vi "Quiz3.vi"() -> ()   [LabVIEW 2019]
panel:
  in  "Tab Control":enum32{"User", "Admi", "DeBug"}(tab)
  out "Gráfica temperatura":dbl(graph)=50.42767726953025
  in  "Temp Max":dbl
  in  "Temp Min":dbl
  out "Alerta":string
  out "Temp Mínima":dbl
  out "Temp máxima":dbl
  in  "Temperatura C":dbl
  out "Temperatura C.":string
  out "Resistencia NTC":dbl
  out "Voltaje":dbl
  out "Temperatura F.":string="-459,670000"
  in  "TIEMPO DE GRAFIACIÓN":dbl
  in  "ALMACENAR CADA Y TIME":dbl
  in  "ADQUIRIR CADA X TIME":dbl
  in  "Escribir Warnings":bool
  in  "Escribir todos lo datos":bool
  in  "MANUAL":bool
  in  "STOP":bool=TRUE
  in  "INICIO":bool=TRUE
  out "Alerta.":string
  out "Gráfica temperatura 3":dbl(graph)=50.42767726953025
  in  "Tab  control graficas":enum32{"Datos ", "Warnings", "Gráfica"}(tab)
  in  "Datos":i32(listbox)
  in  "Warnings":i32(listbox)
  out "Gráfica temperatura 2":dbl(graph)=50.42767726953025
  out "Temperatura °C":string="-273,150000"
  out "ALERTA":string
  # "°C"
  # "°F"
  # "Ohms"
  # "V"
  # "sg"
  # "sg"
  # "sg"
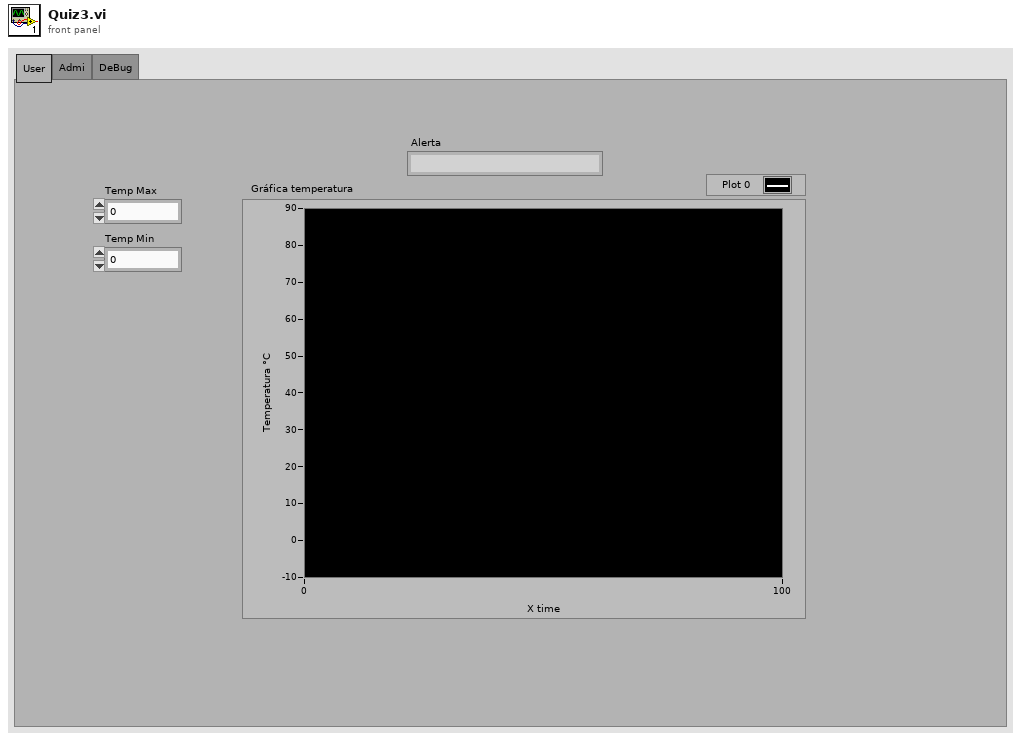
[diagram p1: front panel]
types:
  T1 = cluster{" Grados Cent.":string, "Grados Fare.":string, "date/time string":string, "Nombre del archivo txt":string}
  T2 = cluster{"Temperatura C.":string, "date/time string":string, string, "Nombre del archivo txt":string}
  T3 = cluster{" Grados Cent.":string, "Grados Fare.":string, "date/time string":string, "Nombre del archivo txt":string}[]
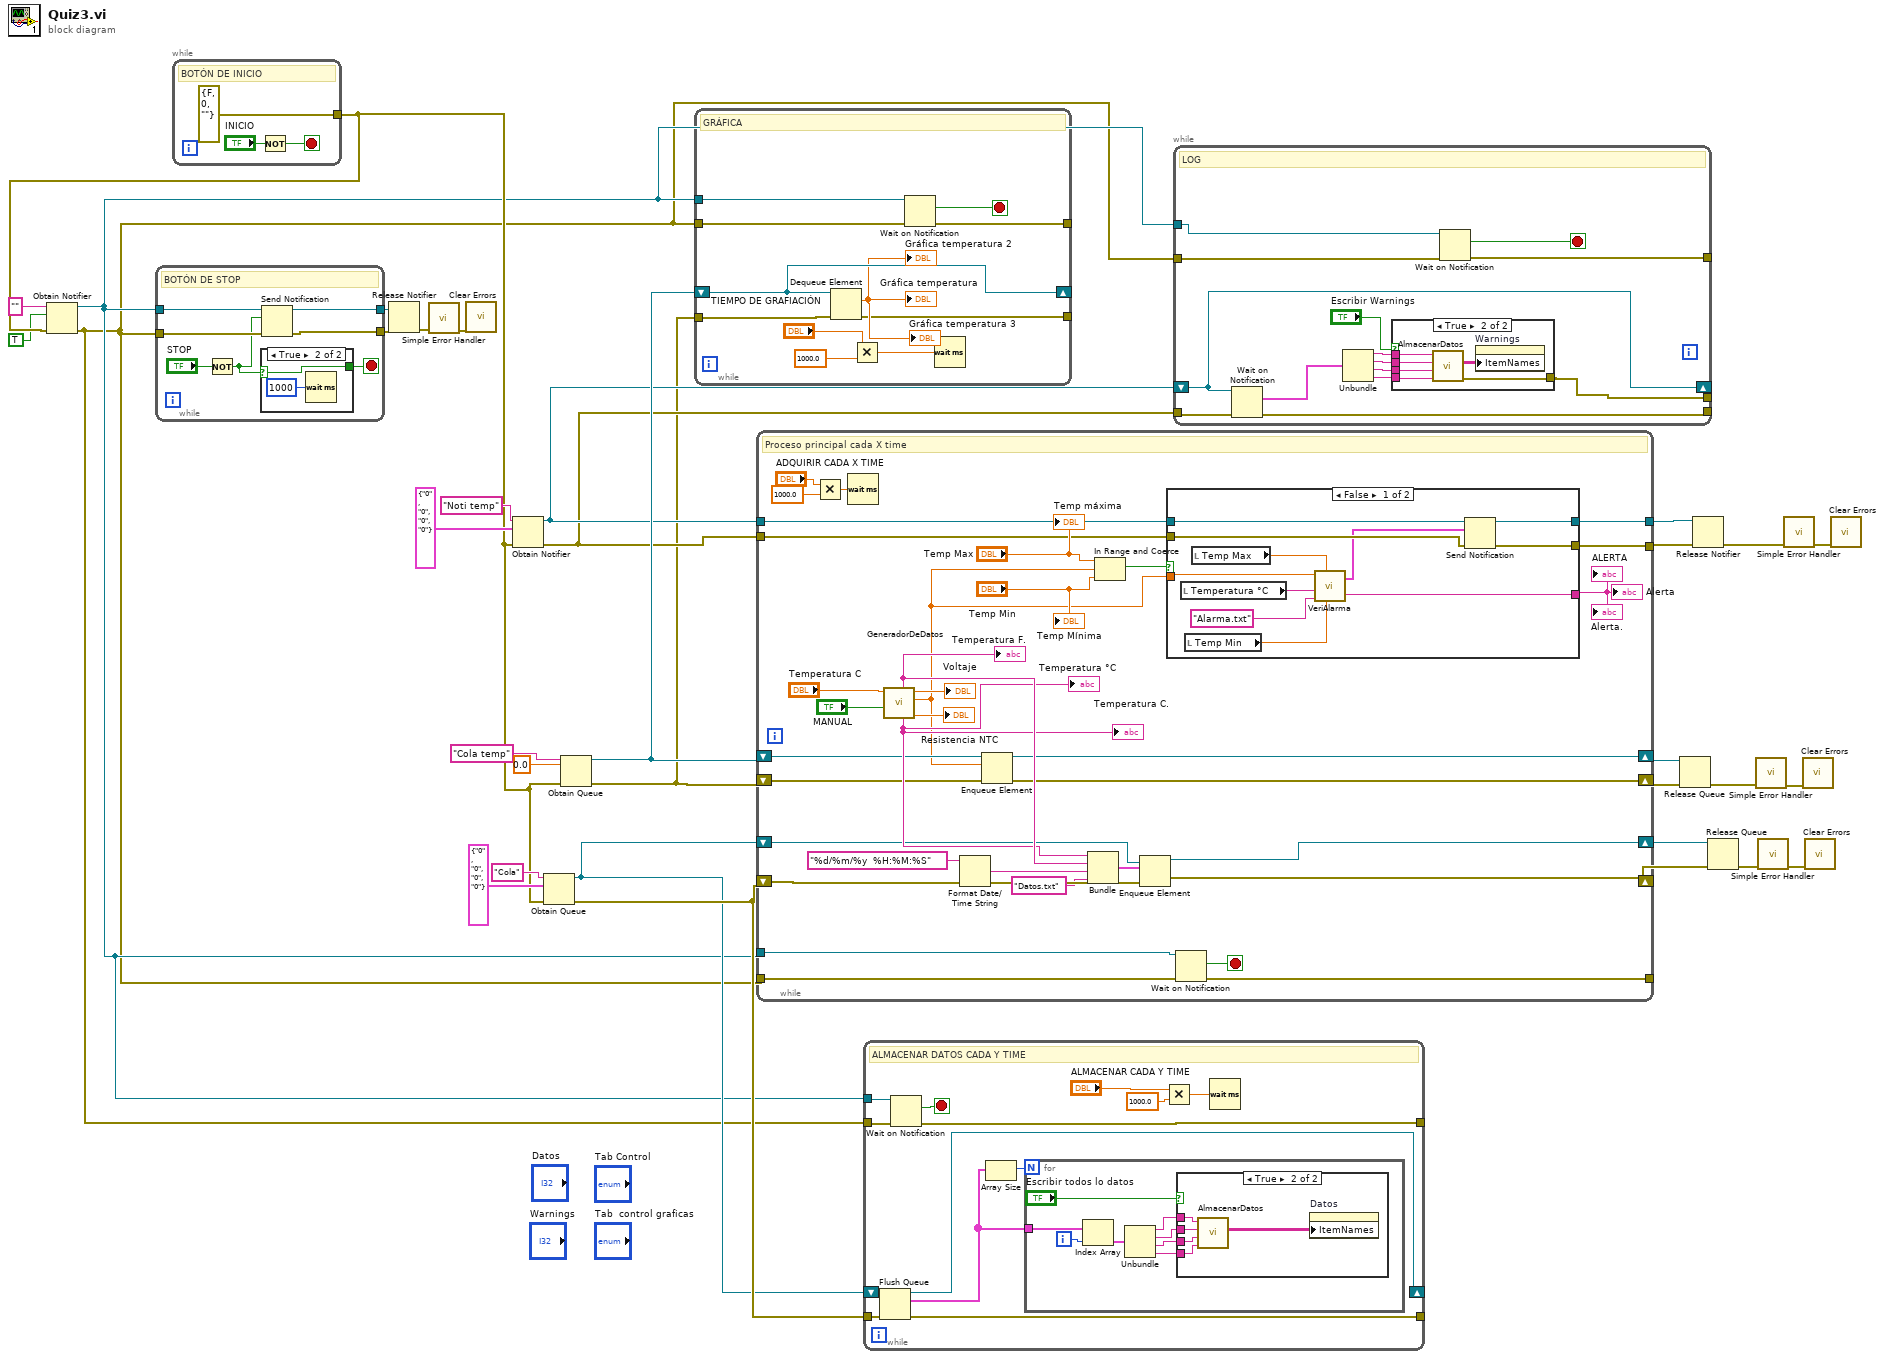
[diagram p0: block diagram]
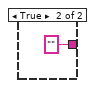
[diagram p5: hidden frame]
diagram:
  n1 = while {
    tunnel: [errorcluster {"status"=FALSE, "code"=0, "source"=""} ("error in (no error)")] -> w10
    stop <- w35 stop-if-true
    # "BOTÓN DE INICIO"
    n2 = Not(x="INICIO") -> (.not. x?=w35:bool)
  }
  n3 = Obtain Notifier(name (unnamed)="", notification data type=TRUE, error in (no error)=w10) -> (notifier out=w2:refnum<notifier>, error out=w1:errorcluster)  [unwired: 1 in, 1 out]
  n4 = while {
    tunnel: w2 -> [w42]
    tunnel: w1 -> [w41]
    tunnel: [w40] -> w6
    tunnel: [w39] -> w4
    stop <- w37 stop-if-true
    # "BOTÓN DE STOP"
    n5 = Not(x="STOP") -> (.not. x?=w38:bool)
    n6 = case shown="True" w38 {
      selector: w38 -> [_ w44]
      tunnel: [_ w44] -> w37
      frame False {
      }
      frame True {
        n7 = Wait (ms)(milliseconds to wait=u32 1000) -> ()  [unwired: 1 out]
      }
    }
    n8 = Send Notification(notification=w38, notifier=w42, error in (no error)=w41) -> (notifier out=w39:refnum<notifier>, error out=w40:errorcluster)
  }
  n9 = Release Notifier(notifier=w4, error in (no error)=w6) -> (error out=w7:errorcluster)  [unwired: 1 in, 2 out]
  n10 = call <vilib>:"Simple Error Handler.vi"("error in (no error)"=w7) -> ("error out"=w5:errorcluster)  [unwired: 4 in, 4 out]
  n11 = call <vilib>:"Clear Errors.vi"("error in (no error)"=w5) -> ()  [unwired: 5 in, 2 out]
  n12 = Obtain Notifier(name (unnamed)="Noti temp", notification data type=T1 {" Grados Cent."="0", "Grados Fare."="0", "date/time string"="0", "Nombre del archivo txt"="0"} ("output cluster"), error in (no error)=w10) -> (notifier out=w21:refnum<notifier>, error out=w20:errorcluster)  [unwired: 1 in, 1 out]
  n13 = Obtain Queue(name (unnamed)="Cola", element data type=T1 {" Grados Cent."="0", "Grados Fare."="0", "date/time string"="0", "Nombre del archivo txt"="0"} ("output cluster"), error in (no error)=w10) -> (queue out=w17:refnum<queue>, error out=w32:errorcluster)  [unwired: 2 in, 1 out]
  n14 = Obtain Queue(name (unnamed)="Cola temp", element data type=0.0, error in (no error)=w10) -> (queue out=w25:refnum<queue>, error out=w3:errorcluster)  [unwired: 2 in, 1 out]
  n15 = while {
    shift-right: [w56] -> _
    shift-left: w25 -> [w56]
    tunnel: w2 -> [w51]
    tunnel: w1 -> [w50]
    tunnel: w3 -> [w49]
    tunnel: [w48] -> _
    tunnel: [w46] -> _
    stop <- w47 stop-if-true
    # "GRÁFICA"
    n16 = Dequeue Element(queue=w56, error in (no error)=w49) -> (element=→"Gráfica temperatura" →"Gráfica temperatura 2" →"Gráfica temperatura 3":dbl, error out=w48:errorcluster)  [unwired: 1 in, 2 out]
    n17 = Multiply(x="TIEMPO DE GRAFIACIÓN", y=1000.0) -> (x*y=w54:dbl)
    n18 = Wait on Notification(notifier=w51, error in (no error)=w50) -> (notification=w47:bool, error out=w46:errorcluster)  [unwired: 2 in, 2 out]
    n19 = Wait (ms)(milliseconds to wait=w54) -> ()  [unwired: 1 out]
  }
  n20 = while {
    shift-right: [w78] -> w31
    shift-left: w17 -> [w82]
    shift-right: [w62] -> w30
    shift-left: w32 -> [w81]
    shift-right: [w75] -> w27
    shift-left: w25 -> [w77]
    shift-right: [w63] -> w26
    shift-left: w3 -> [w76]
    tunnel: w21 -> [w71]
    tunnel: [w69] -> w23
    tunnel: w20 -> [w70]
    tunnel: [w68] -> w22
    tunnel: w2 -> [w60]
    tunnel: w1 -> [w59]
    tunnel: [w57] -> _
    stop <- w58 stop-if-true
    # "Proceso principal cada X time"
    n21 = Multiply(x="ADQUIRIR CADA X TIME", y=1000.0) -> (x*y=w64:dbl)
    n22 = Wait (ms)(milliseconds to wait=w64) -> ()  [unwired: 1 out]
    n23 = call "GeneradorDeDatos.vi"("MANUAL"="MANUAL", "Temp"="Temperatura C") -> ("NTC"=→"Resistencia NTC":dbl, "Grados C graf"=w67:dbl, "Voltaje"=→"Voltaje":dbl, "Grados Cent."=w87:string, "Grados Fare."=w88:string)  [unwired: 5 in]
    "Temperatura C." <- w87
    "Temperatura F." <- w88
    "Temperatura °C" <- w87
    n24 = Format Date/Time String(time format string (%c)="%d/%m/%y  %H:%M:%S") -> (date/time string=w89:string)  [unwired: 2 in]
    n25 = Enqueue Element(queue=w77, element=w67, error in (no error)=w76) -> (queue out=w75:refnum<queue>, error out=w63:errorcluster)  [unwired: 1 in, 1 out]
    n26 = Bundle("Grados Cent."=w87, "Grados Fare."=w88, "date/time string"=w89, "Nombre del archivo txt"="Datos.txt") -> (w90:T1)  [unwired: 1 in]
    n27 = In Range and Coerce(upper limit="Temp Max", x=w67, lower limit="Temp Min") -> (In Range?=w72:bool)  [unwired: 1 out]
    n28 = Enqueue Element(queue=w82, element=w90, error in (no error)=w81) -> (queue out=w78:refnum<queue>, error out=w62:errorcluster)  [unwired: 1 in, 1 out]
    n29 = case shown="False" w72 {
      tunnel: w71 -> [w101 _]
      tunnel: w70 -> [w100 _]
      tunnel: [w99 _] -> w69
      tunnel: [w98 _] -> w68
      tunnel: w67 -> [w91 _]
      tunnel: [w96 ""] -> w66
      frame False {
        n30 = local read "Temperatura °C"() -> (w93:string)
        n31 = local read "Temp Min"() -> (w94:dbl)
        n32 = local read "Temp Max"() -> (w95:dbl)
        n33 = call "VeriAlarma.vi"("Temp Min"=w94, "Temp Max"=w95, "Nombre del archivo txt"="Alarma.txt", "Temp grados C"=w93, "Grados C"=w91) -> ("Alarma"=w96:string, "Notify Datos"=w97:T2)  [unwired: 1 in]
        n34 = Send Notification(notification=w97, notifier=w101, error in (no error)=w100) -> (notifier out=w99:refnum<notifier>, error out=w98:errorcluster)
      }
      frame True {
      }
    }
    "Alerta" <- w66
    "ALERTA" <- w66
    "Alerta." <- w66
    n35 = Wait on Notification(notifier=w60, error in (no error)=w59) -> (notification=w58:bool, error out=w57:errorcluster)  [unwired: 2 in, 2 out]
    "Temp Mínima" <- "Temp Min"
    "Temp máxima" <- "Temp Max"
  }
  n36 = while {
    shift-right: [w111] -> _
    shift-left: w17 -> [w112]
    tunnel: w32 -> [w108]
    tunnel: w2 -> [w107]
    tunnel: w1 -> [w106]
    tunnel: [w105] -> _
    tunnel: [w103] -> _
    stop <- w104 stop-if-true
    # "ALMACENAR DATOS CADA Y TIME"
    n37 = Flush Queue(queue=w112, error in (no error)=w108) -> (queue out=w111:refnum<queue>, remaining elements=w109:T3, error out=w105:errorcluster)
    n38 = Wait on Notification(notifier=w107, error in (no error)=w106) -> (notification=w104:bool, error out=w103:errorcluster)  [unwired: 2 in, 2 out]
    n39 = Array Size(array=w109) -> (size(s)=w110:i32)
    n40 = for {
      N: w110 -> [_]
      tunnel: w109 -> [w122]
      i -> [w123]
      n41 = Index Array(array=w122, index=w123) -> (element=w116:T1)
      n42 = Unbundle(w116) -> ("Grados Cent."=w117:string, "Grados Fare."=w118:string, "date/time string"=w119:string, "Nombre del archivo txt"=w120:string)
      n43 = case shown="True" "Escribir todos lo datos" {
        tunnel: w117 -> [_ w128]
        tunnel: w118 -> [_ w127]
        tunnel: w119 -> [_ w126]
        tunnel: w120 -> [_ w125]
        frame False {
        }
        frame True {
          n44 = call "AlmacenarDatos.vi"("Nombre del archivo txt"=w125, "StampTime"=w126, "Fare."=w127, "Cent"=w128) -> ("all rows"=w124:string[][])  [unwired: 6 in, 1 out]
          n45 = property on="Datos" class="MCListbox (strict)"("ItemNames"=w124) -> ()  [unwired: 2 in, 2 out]
        }
      }
    }
    n46 = Multiply(x="ALMACENAR CADA Y TIME", y=1000.0) -> (x*y=w113:dbl)
    n47 = Wait (ms)(milliseconds to wait=w113) -> ()  [unwired: 1 out]
  }
  n48 = while {
    tunnel: w20 -> [w142]
    shift-right: [w136] -> _
    shift-left: w21 -> [w136]
    tunnel: [w134] -> _
    tunnel: [w133] -> _
    tunnel: [w132] -> _
    tunnel: w2 -> [w131]
    tunnel: w1 -> [w130]
    stop <- w129 stop-if-true
    # "LOG"
    n49 = Wait on Notification(notifier=w136, error in (no error)=w142) -> (notification=w141:T1, error out=w133:errorcluster)  [unwired: 2 in, 2 out]
    n50 = Unbundle(w141) -> ("Grados Cent."=w140:string, "Grados Fare."=w139:string, "date/time string"=w138:string, "Nombre del archivo txt"=w137:string)
    n51 = case shown="True" "Escribir Warnings" {
      tunnel: w140 -> [_ w148]
      tunnel: w139 -> [_ w147]
      tunnel: w138 -> [_ w146]
      tunnel: w137 -> [_ w145]
      tunnel: [_ w143] -> w134
      frame False {
      }
      frame True {
        n52 = call "AlmacenarDatos.vi"("Nombre del archivo txt"=w145, "StampTime"=w146, "Fare."=w147, "Cent"=w148) -> ("error out"=w143:errorcluster, "all rows"=w144:string[][])  [unwired: 6 in]
        n53 = property on="Warnings" class="MCListbox (strict)"("ItemNames"=w144) -> ()  [unwired: 2 in, 2 out]
      }
    }
    n54 = Wait on Notification(notifier=w131, error in (no error)=w130) -> (notification=w129:bool, error out=w132:errorcluster)  [unwired: 2 in, 2 out]
  }
  n55 = Release Queue(queue=w27, error in (no error)=w26) -> (error out=w13:errorcluster)  [unwired: 1 in, 2 out]
  n56 = Release Notifier(notifier=w23, error in (no error)=w22) -> (error out=w16:errorcluster)  [unwired: 1 in, 2 out]
  n57 = Release Queue(queue=w31, error in (no error)=w30) -> (error out=w11:errorcluster)  [unwired: 1 in, 2 out]
  n58 = call <vilib>:"Simple Error Handler.vi"("error in (no error)"=w13) -> ("error out"=w14:errorcluster)  [unwired: 4 in, 4 out]
  n59 = call <vilib>:"Simple Error Handler.vi"("error in (no error)"=w11) -> ("error out"=w12:errorcluster)  [unwired: 4 in, 4 out]
  n60 = call <vilib>:"Simple Error Handler.vi"("error in (no error)"=w16) -> ("error out"=w15:errorcluster)  [unwired: 4 in, 4 out]
  n61 = call <vilib>:"Clear Errors.vi"("error in (no error)"=w14) -> ()  [unwired: 5 in, 2 out]
  n62 = call <vilib>:"Clear Errors.vi"("error in (no error)"=w12) -> ()  [unwired: 5 in, 2 out]
  n63 = call <vilib>:"Clear Errors.vi"("error in (no error)"=w15) -> ()  [unwired: 5 in, 2 out]
